vi "Stop Core.vi"(10 "final error code":i32, 11 "Form Model in":refnum<class "Form Model.lvclass">) -> (3 "Form Model out":refnum<class "Form Model.lvclass">)   [LabVIEW 2020, in "Form Model.lvlib" / "Form Model.lvclass"]
doc: "(<B>Filename</B>: Actor Framework.lvlib:Actor.lvclass:Stop Core.vi)\n\nDefines what the actor does before it stops. Use the <B>final error code</B> input to determine whether the actor shut down in response to an error.\n\nBy default, this method passes the Stop message along to all auto-stop nested actors. A descendant class may override this method to define additional behavior, such as shutting down any processes the actor initiated in its override of the Actor Core method."
uses:
  Form Model.lvclass
  C:/Program Files (x86)/National Instruments/LabVIEW 2020/vi.lib/ActorFramework/Actor/Actor.lvclass
  <vilib>/ActorFramework/Actor/Actor.lvclass/Actor.ctl
  Form Model.lvclass/Form Model.ctl
  Form Server Messages Messages/Close Form Msg/Close Form Msg.lvclass/Close Form Msg.ctl
  <vilib>/ActorFramework/Message Enqueuer/Message Enqueuer.lvclass/Message Enqueuer.ctl
  <vilib>/ActorFramework/Message Enqueuer/Enqueue.vi
  Form Server Messages Messages/Close Form Msg/Close Form Msg.lvclass
  C:/Program Files (x86)/National Instruments/LabVIEW 2020/vi.lib/ActorFramework/Message/Message.lvclass
  <vilib>/ActorFramework/Message Priority Queue/Priority Enqueue.vi
  <vilib>/MGI/Monitored Actor/Monitored Actor/Monitored Actor/Monitored Actor.lvclass
  Form Configuration/Form Configuration.lvclass
  <vilib>/ActorFramework/Actor/Actor.lvclass
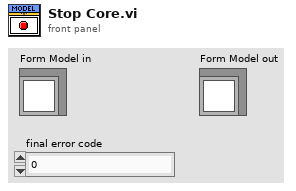
[diagram p1: front panel]
types:
  T1 = typedef "Form Server Interfaces.lvlib/Form ID.ctl" = cluster{"Name":string, "Panel type":string}
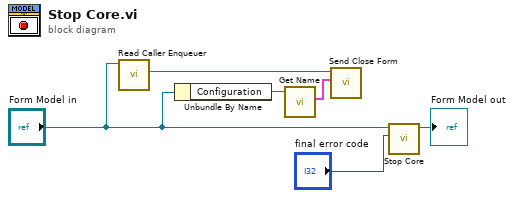
[diagram p0: block diagram]
diagram:
  n1 = call <vilib>:"Read Caller Enqueuer.vi"("Actor"="Form Model in") -> ("Caller Enqueuer"=w4:refnum<class "Message Enqueuer.lvclass">)  [unwired: 10 in]
  n2 = Unbundle By Name("Form Model in") -> ("Configuration"=w2:refnum<class "Form Configuration.lvclass">)
  n3 = call-dynamic "Get Name.vi"("Form Configuration in"=w2) -> ("Form ID"=w1:T1)  [unwired: 8 in, 2 out]
  n4 = call "Send Close Form.vi"("Form Name"=w1, "Message Enqueuer"=w4) -> ()  [unwired: 8 in, 2 out]
  n5 = call-parent "Stop Core.vi"("final error code"="final error code", "Monitored Actor in"="Form Model in") -> ("Monitored Actor out"=→"Form Model out":refnum<class "Form Model.lvclass">)  [unwired: 9 in]
